vi "example_agent_example_sm_template.vi"() -> ()   [LabVIEW 2020]
uses:
  src/user_interfaces/simple_html_chat_ui/simple_html_chat_ui.lvclass
  src/models/abstract_llm_base/abstract_llm_base.lvclass
  src/vectorstore/abstract_vector_base/abstract_vector_base.lvclass
  src/agent/agent_simple_qa/agent_simple_qa.lvclass
  src/models/message_text/message_text.lvclass
  <vilib>/addons/_JKI Toolkits/State Machine/_JKI_lib_State_Machine.llb/Select State(s)_err__jki_lib_state_machine.vi
  src/vectorstore/vector_qdrant/vector_qdrant.lvclass
  C:/LV_LLM/src/vectorstore/abstract_vector_base/abstract_vector_base.lvclass
  src/models/llm_openai_chatmodels/llm_openai_chatmodels.lvclass
  C:/LV_LLM/src/models/abstract_llm_base/abstract_llm_base.lvclass
  src/models/llm_openai_embedding/llm_openai_embedding.lvclass
  src/agent/agent_simple_qa_dynamicdata/agent_simple_qa_dynamic.lvclass
  C:/LV_LLM/src/agent/agent_simple_qa/agent_simple_qa.lvclass
  <vilib>/addons/_JKI Toolkits/State Machine/_JKI_lib_State_Machine.llb/Periodic Trigger__ogtk__JKI-SM__jki_lib_state_machine.vi
  src/models/message_text/create_text_message.vi
  src/models/message_text/create_error_message.vi
  src/models/llm_openai_chatmodels/Instantiate_llm_openai.vi
  src/models/llm_openai_embedding/Instantiate_llm_openai_embed.vi
  src/agent/agent_simple_qa/poly/ask_your_data.vi
panel:
  in  "Simulate Error":bool
  in  "new_message":string
  in  "send":bool
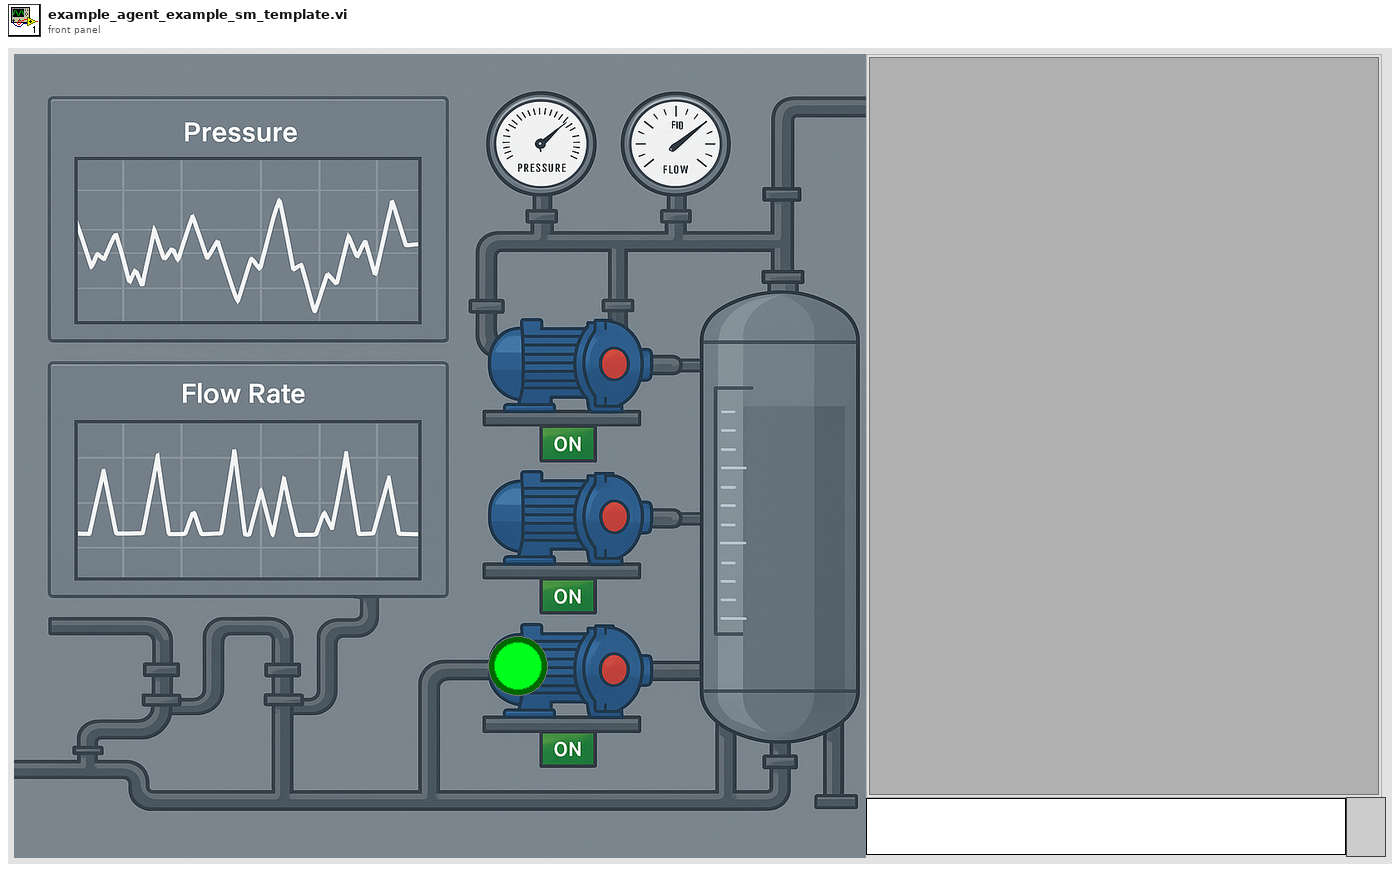
[diagram p1: front panel]
types:
  T1 = enum32{"Invalid", "Standard", "Closed", "Hidden", "Minimized", "Maximized"}
  T2 = enum32{"invalid app kind", "Development System", "Run Time System", "Student Edition", "Embedded LabVIEW", "Evaluation", "Custom"}
  T3 = cluster{"Core":cluster{"Current VI Reference":refnum<vi>, "Close Panel on Exit?":bool}, "Agent":cluster{"UI_Chat":refnum<class "simple_html_chat_ui.lvclass">, "Model_Generative":refnum<class "abstract_llm_base.lvclass">, "Model_Embedding":refnum<class "abstract_llm_base.lvclass">, "Vector Store":refnum<class "abstract_vector_base.lvclass">, "Agent_QA":refnum<class "agent_simple_qa.lvclass">, "last_message":refnum<class "message_text.lvclass">}}
  T4 = cluster{"UI_Chat":refnum<class "simple_html_chat_ui.lvclass">, "Model_Generative":refnum<class "abstract_llm_base.lvclass">, "Model_Embedding":refnum<class "abstract_llm_base.lvclass">, "Vector Store":refnum<class "abstract_vector_base.lvclass">, "Agent_QA":refnum<class "agent_simple_qa.lvclass">, "last_message":refnum<class "message_text.lvclass">}
  T5 = cluster{"Current VI Reference":refnum<vi>, "Close Panel on Exit?":bool}
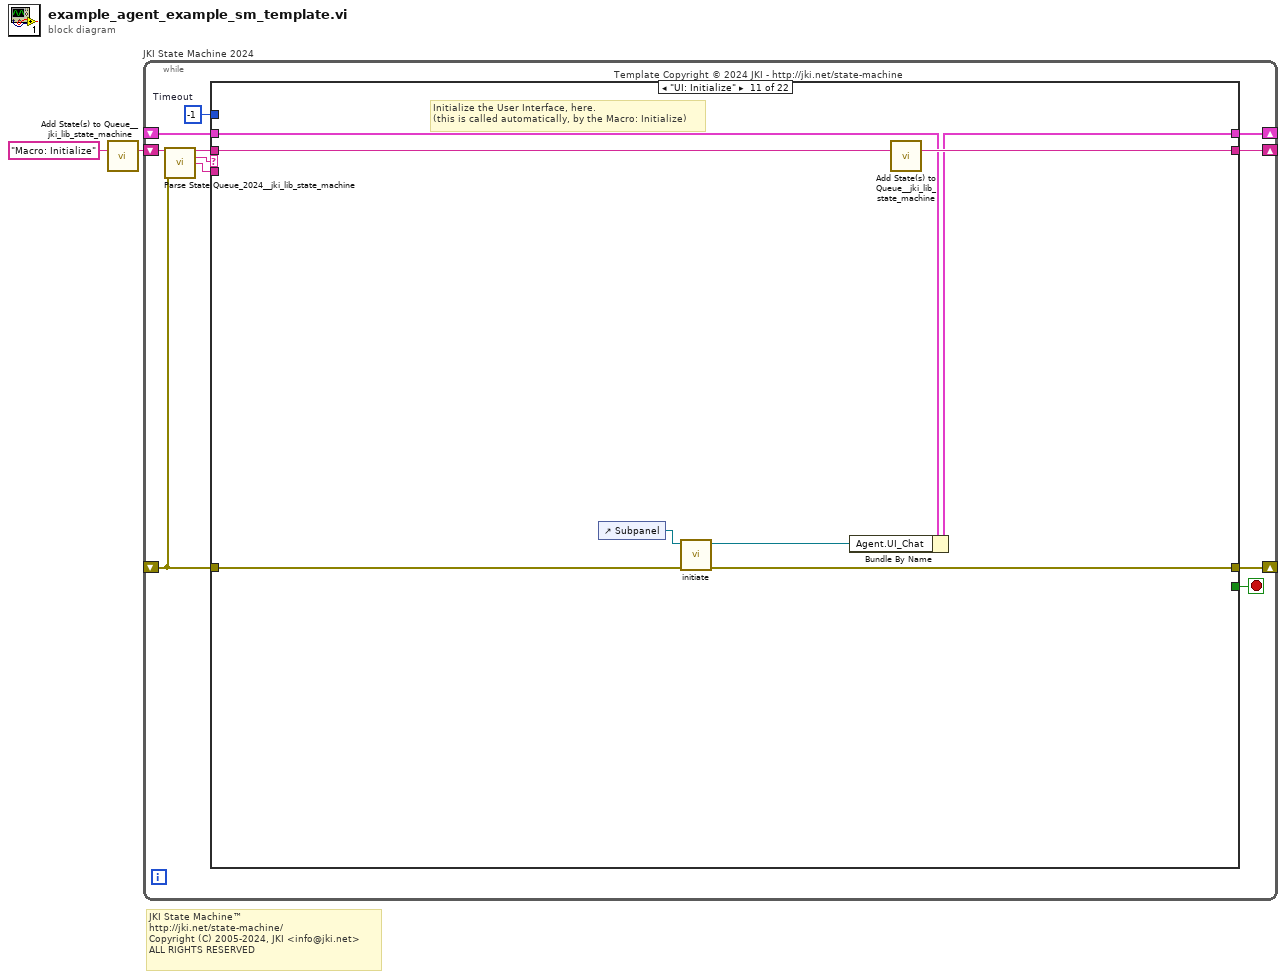
[diagram p0: block diagram]
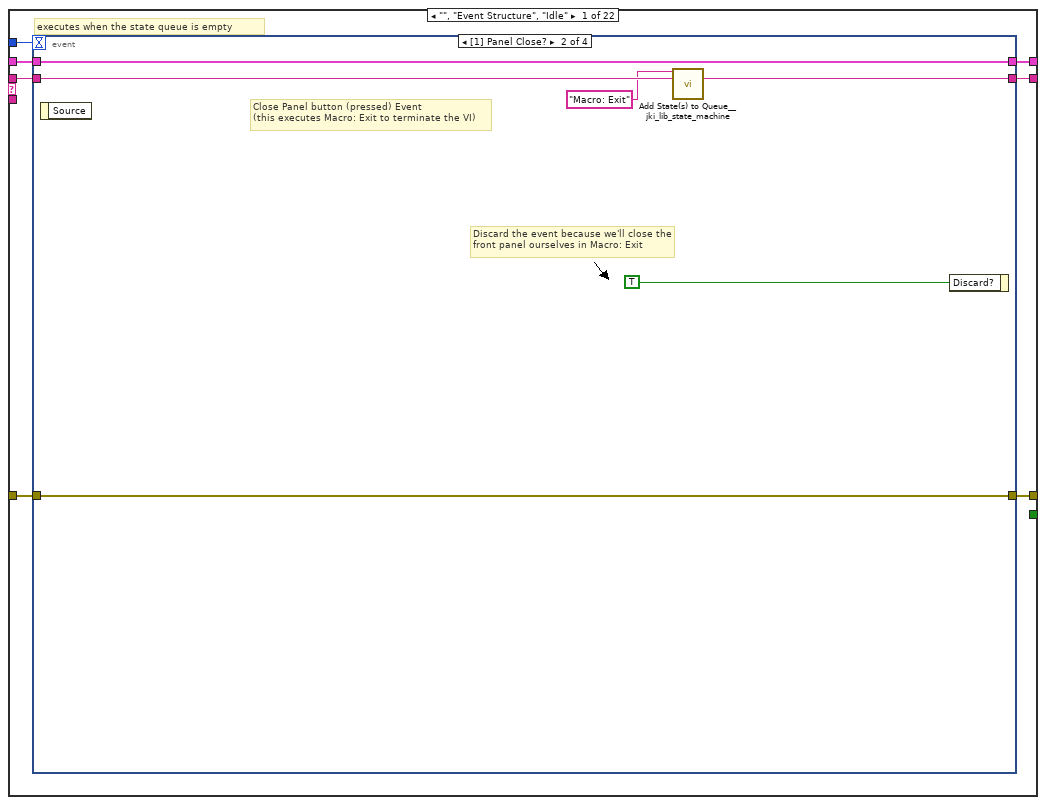
[diagram p2: hidden frame]
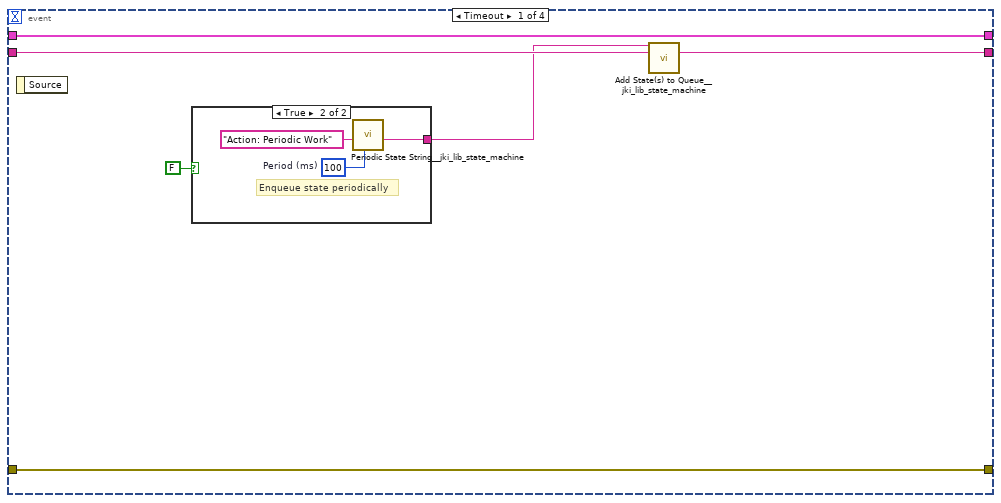
[diagram p3: hidden frame]
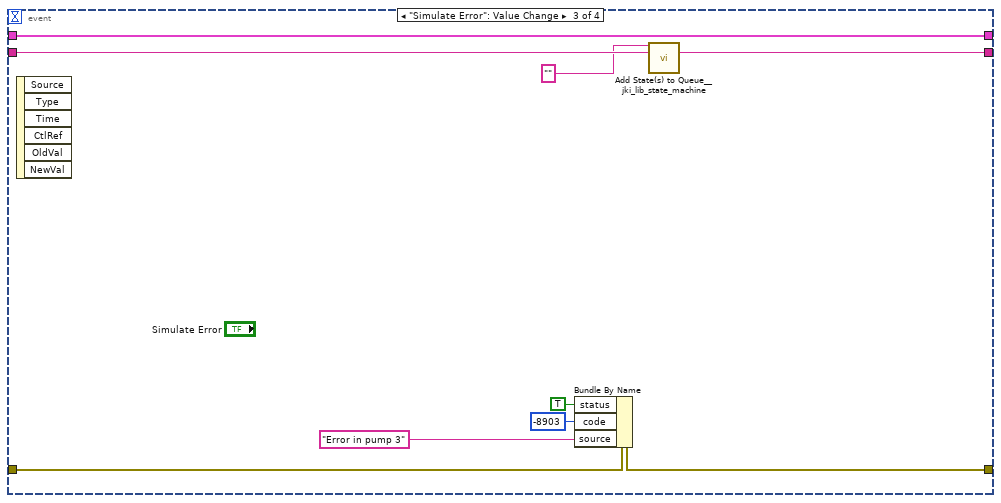
[diagram p5: hidden frame]
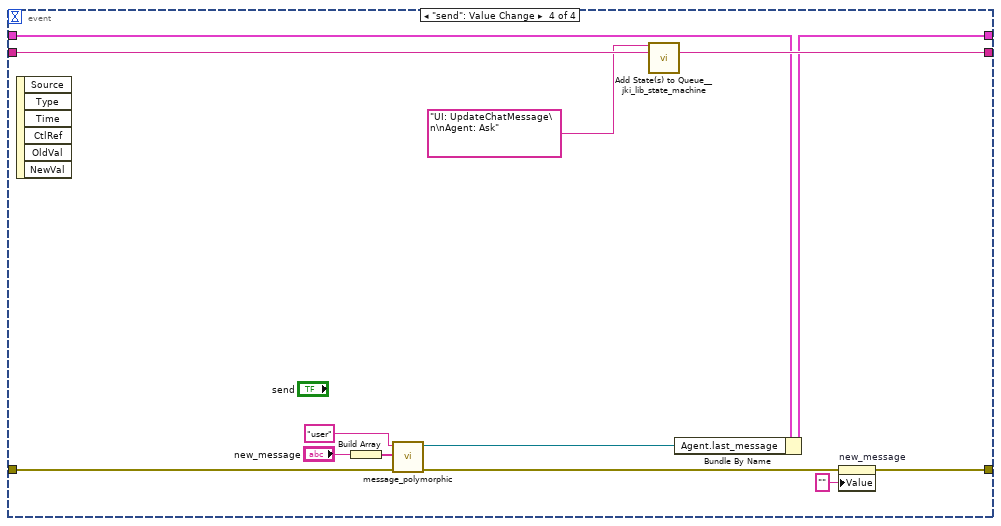
[diagram p6: hidden frame]
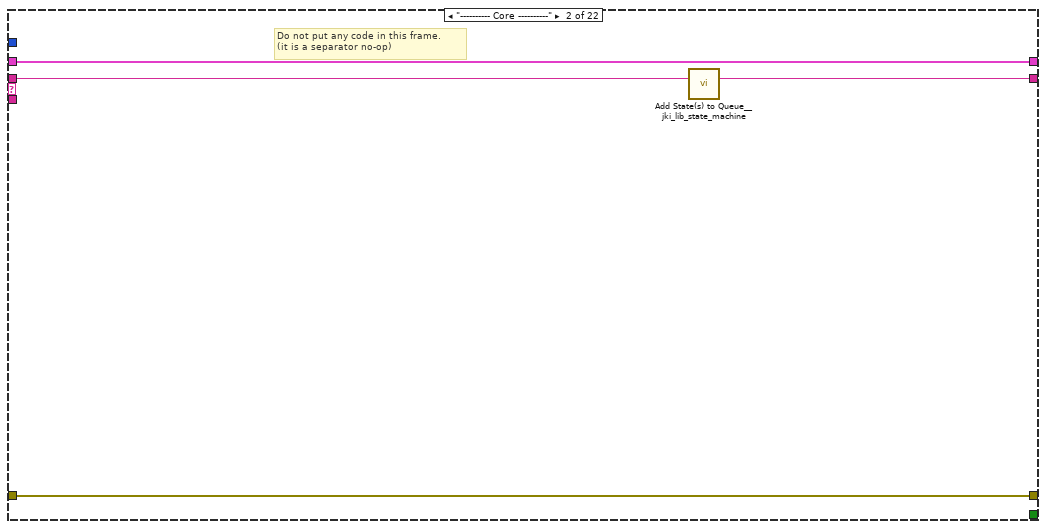
[diagram p7: hidden frame]
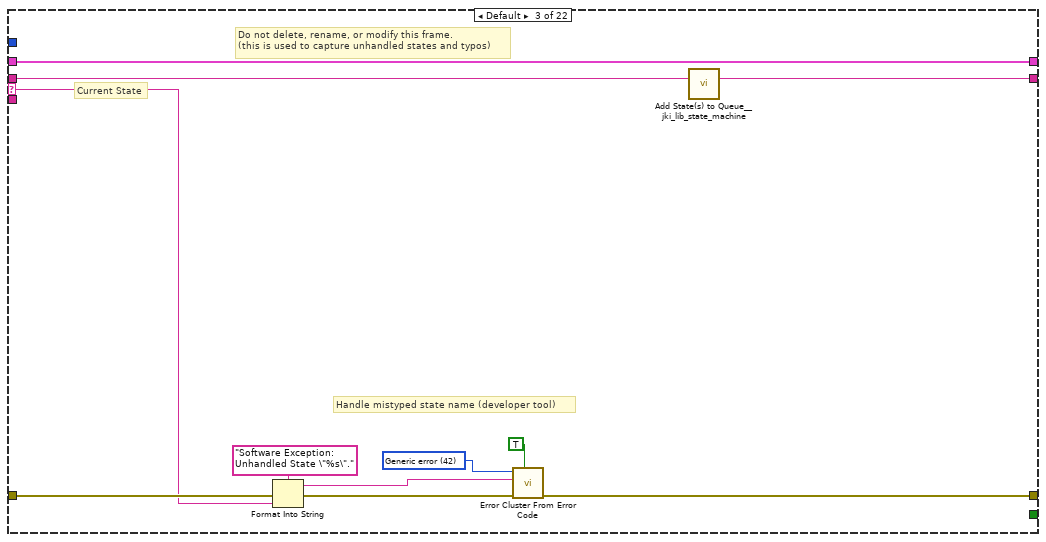
[diagram p8: hidden frame]
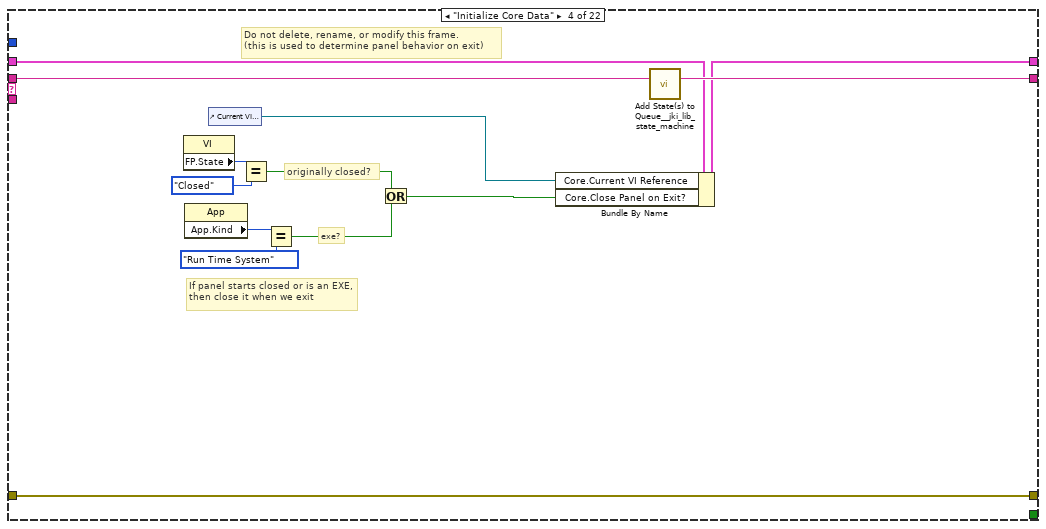
[diagram p9: hidden frame]
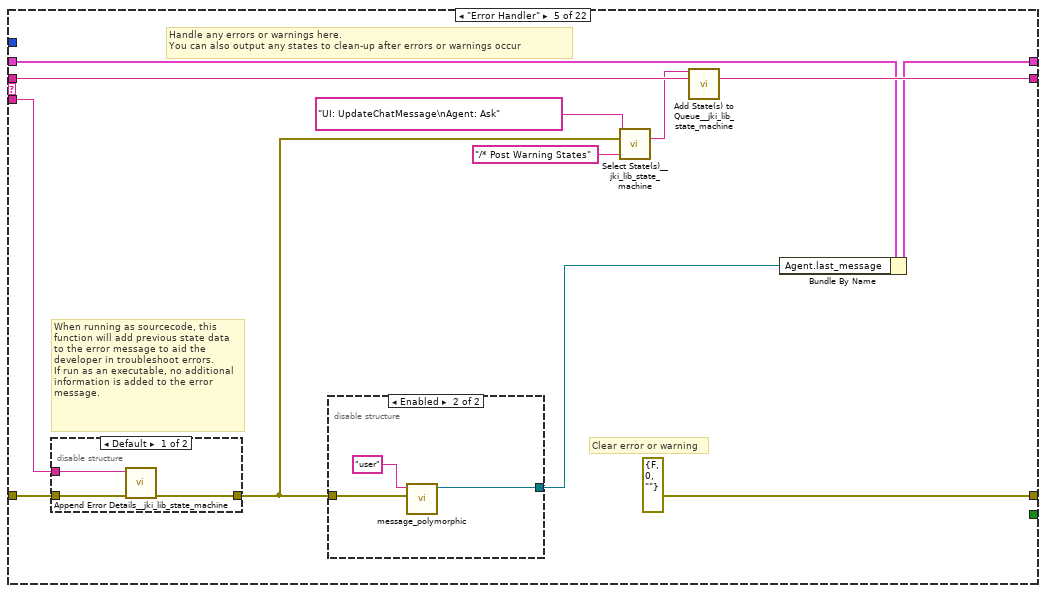
[diagram p10: hidden frame]
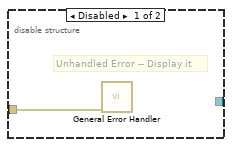
[diagram p11: hidden frame]
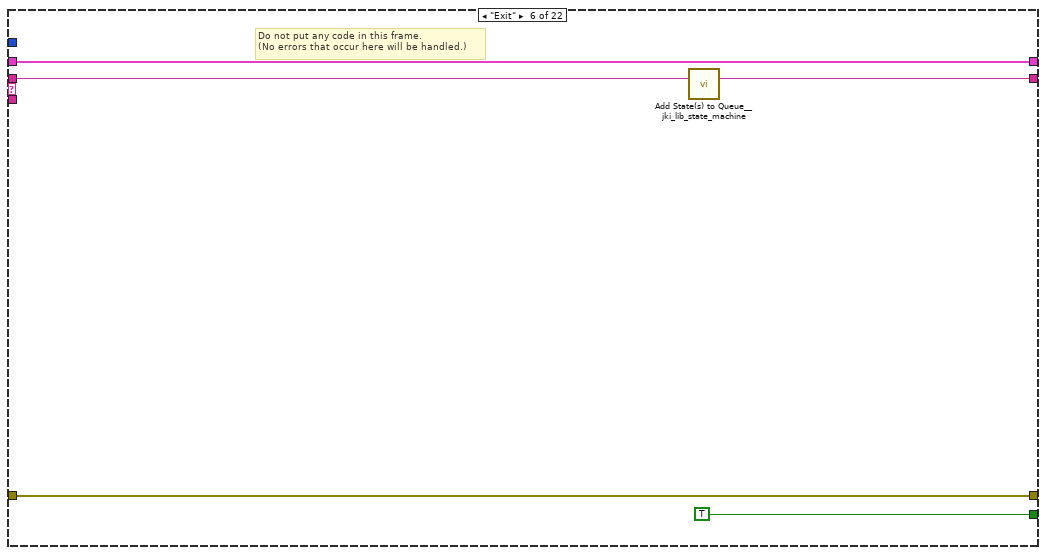
[diagram p13: hidden frame]
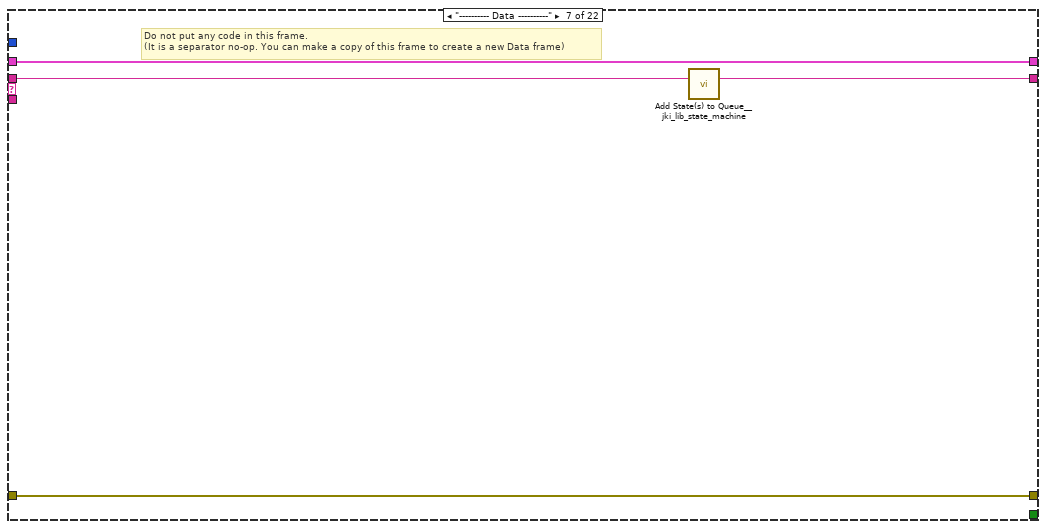
[diagram p14: hidden frame]
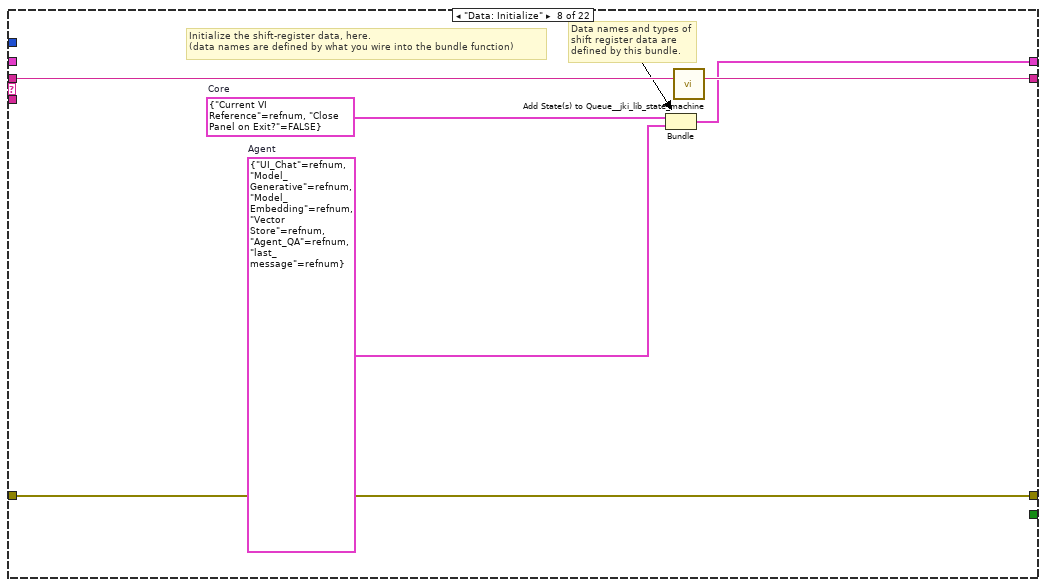
[diagram p15: hidden frame]
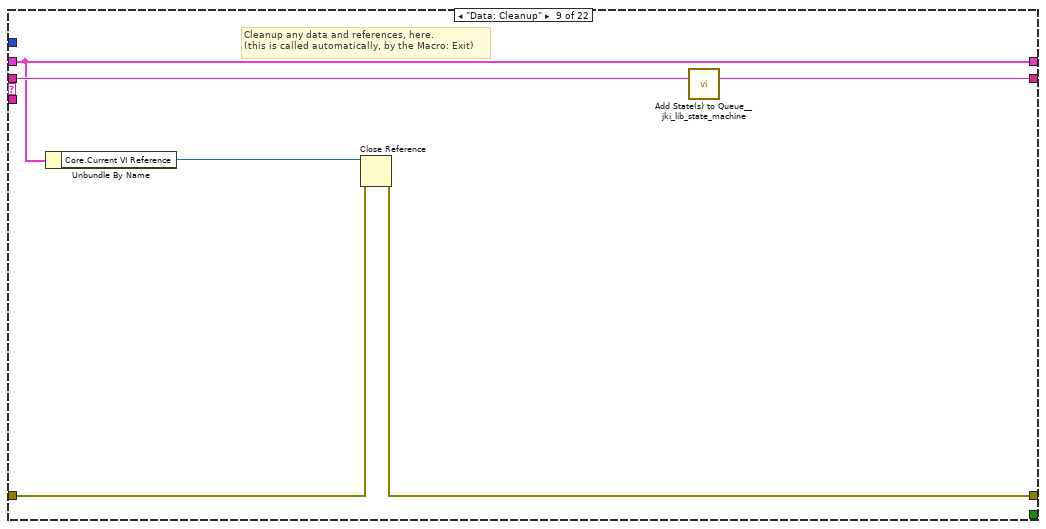
[diagram p16: hidden frame]
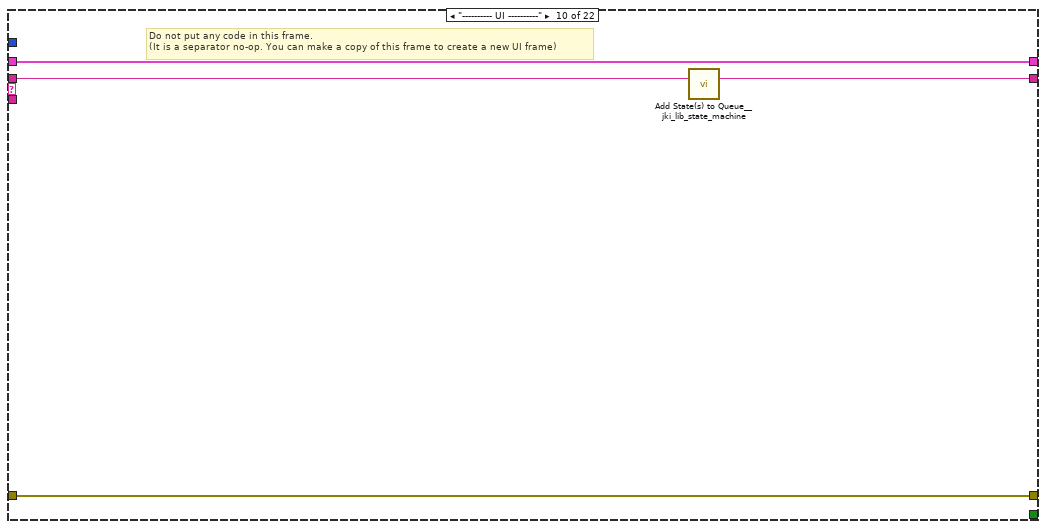
[diagram p17: hidden frame]
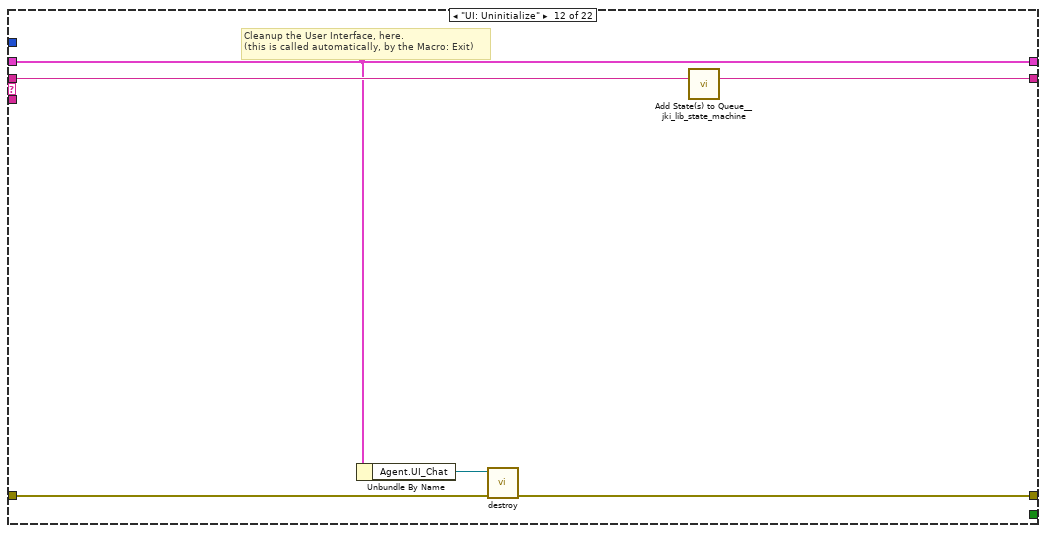
[diagram p18: hidden frame]
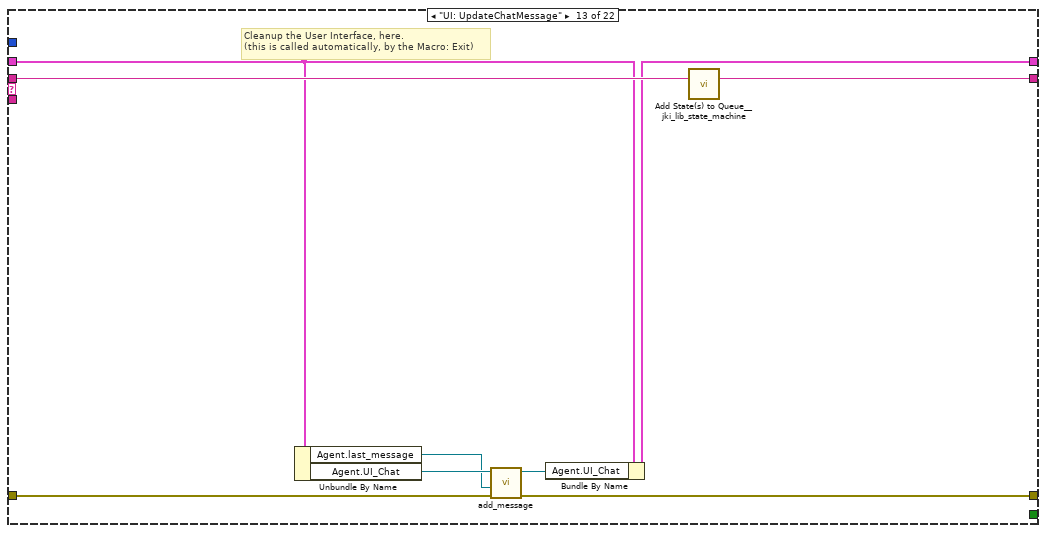
[diagram p19: hidden frame]
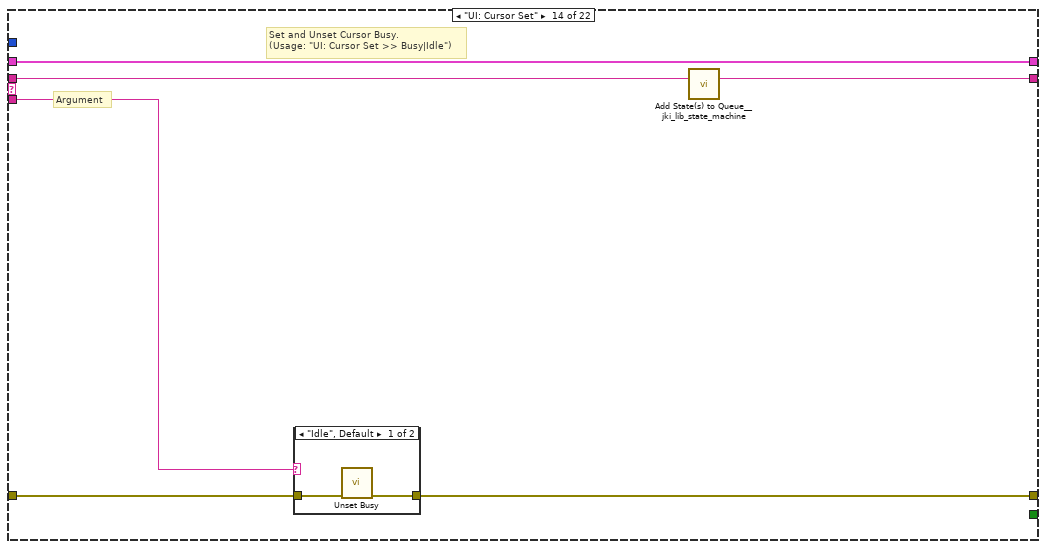
[diagram p20: hidden frame]
diagram:
  # "JKI State Machine™\nhttp://jki.net/state-machine/\nCopyright (C) 2005-2024, JKI <info@jki.net>\nALL RIGHTS RESERVED"
  n1 = call <vilib>:"Add State(s) to Queue__jki_lib_state_machine.vi"("State(s) in (\"\")"="Macro: Initialize") -> ("States Out"=w2:string)  [unwired: 14 in]
  n2 = while "JKI State Machine 2024" {
    shift-right: [w6] -> _
    shift-left: _ -> [w5]
    shift-right: [w9] -> _
    shift-left: _ -> [w3]
    shift-right: [w8] -> _
    shift-left: w2 -> [w10]
    stop <- w7 stop-if-true
    w4 = -1  # Timeout
    # "Template Copyright © 2024 JKI - http://jki.net/state-machine"
    n3 = call <vilib>:"Parse State Queue_2024__jki_lib_state_machine.vi"("State Queue"=w10, "Error In (no error)"=w3) -> ("Remaining States"=w12:string, "Current State"=w13:string, "Arguments"=w11:string)  [unwired: 11 in]
    n4 = case shown="\"UI: Initialize\"" w13 {
      selector: w13 -> [_ _ w62 _ _ _ _ _ _ _ _ _ _ _ _ _ _ _ _ _ _ _]
      tunnel: w12 -> [w20 w61 w66 w85 w97 w110 w114 w120 w126 w130 w138 w144 w153 w159 w170 w239 w244 w253 w257 w281 w293 w304]
      tunnel: w11 -> [_ _ _ _ w93 _ _ _ _ _ _ _ _ w154 w164 _ _ _ _ _ _ _]
      tunnel: w5 -> [w18 w58 w64 w78 w88 w108 w111 _ w121 w127 w133 w142 w148 w157 w166 w236 w241 w251 w254 w263 w291 w299]
      tunnel: [w17 w59 w68 w82 errorcluster {"status"=FALSE, "code"=0, "source"=""} ("error out") w107 w112 w117 w122 w128 w136 w140 w150 w155 w167 w237 w242 w248 w255 w269 w285 w300] -> w9
      tunnel: w3 -> [w14 w59 w67 w82 w94 w107 w112 w117 w123 w128 w134 w141 w151 w156 w168 w237 w242 w248 w255 w267 w289 w301]
      tunnel: [w19 w60 w65 w84 w96 w109 w113 w119 w125 w129 w137 w143 w152 w158 w169 w238 w243 w252 w256 w280 w292 w303] -> w8
      tunnel: [_ _ _ _ _ TRUE _ _ _ _ _ _ _ _ _ _ _ _ _ _ _ _] -> w7
      tunnel: [w16 w58 w64 w83 w86 w108 w111 w118 w121 w127 w132 w142 w147 w157 w166 w236 w241 w251 w254 w262 w291 w297] -> w6
      tunnel: w4 -> [w15 _ _ _ _ _ _ _ _ _ _ _ _ _ _ _ _ _ _ _ _ _]
      frame "", "Event Structure", "Idle" {
        # "executes when the state queue is empty"
        n5 = event shown="[1] Panel Close?" {
          selector: _ -> [_ _ _ _]
          dyn-events: _ -> [_ _ _ _]
          timeout: w15 -> [_ _ _ _]
          tunnel: w20 -> [w26 w35 w44 w57]
          tunnel: [w25 w34 w43 w56] -> w19
          tunnel: w18 -> [w23 w32 w42 w50]
          tunnel: [w24 w33 w39 w46] -> w17
          tunnel: w14 -> [w24 w33 w40 w52]
          tunnel: [w23 w32 w42 w48] -> w16
          event Timeout {
            n6 = event-data() -> ()  [unwired: 1 in, 1 out]
            n7 = case shown="True" FALSE {
              tunnel: [_ w29] -> w22
              frame False {
              }
              frame True {
                w27 = u32 100  # Period (ms)
                # "Enqueue state periodically"
                n8 = call <vilib>:"Periodic State String__jki_lib_state_machine.vi"("Period (ms)"=w27, "State"="Action: Periodic Work") -> ("State Out"=w29:string)  [unwired: 9 in]
              }
            }
            n9 = call <vilib>:"Add State(s) to Queue__jki_lib_state_machine.vi"("State(s) in Front (\"\")"=w22, "State(s) in (\"\")"=w26) -> ("States Out"=w25:string)  [unwired: 13 in]
          }
          event Panel Close? {
            # "Discard the event because we'll close the front panel ourselves in Macro: Exit"
            # "Close Panel button (pressed) Event\n(this executes Macro: Exit to terminate the VI)"
            n10 = event-data() -> ()  [unwired: 1 in, 1 out]
            n11 = call <vilib>:"Add State(s) to Queue__jki_lib_state_machine.vi"("State(s) in Front (\"\")"="Macro: Exit", "State(s) in (\"\")"=w35) -> ("States Out"=w34:string)  [unwired: 13 in]
            n12 = event-data("Discard?"=TRUE) -> ()  [unwired: 1 in, 1 out]
          }
          event "Simulate Error": Value Change {
            n13 = event-data() -> ()  [unwired: 1 in, 6 out]
            n14 = Bundle By Name(cluster=w40, "status"=TRUE, "code"=-8903, "source"="Error in pump 3") -> (w39:errorcluster)
            n15 = call <vilib>:"Add State(s) to Queue__jki_lib_state_machine.vi"("State(s) in Front (\"\")"="", "State(s) in (\"\")"=w44) -> ("States Out"=w43:string)  [unwired: 13 in]
          }
          event "send": Value Change {
            n16 = event-data() -> ()  [unwired: 1 in, 6 out]
            n17 = Build Array("new_message") -> (w53:string[])
            n18 = call-poly "message_polymorphic.vi"("error in (no error)"=w52, "content"=w53, "role"="user") -> ("error out"=w47:errorcluster, "message_text out"=w49:refnum<class "message_text.lvclass">)  [unwired: 7 in]
            n19 = call <vilib>:"Add State(s) to Queue__jki_lib_state_machine.vi"("State(s) in Front (\"\")"="UI: UpdateChatMessage\n\nAgent: Ask", "State(s) in (\"\")"=w57) -> ("States Out"=w56:string)  [unwired: 13 in]
            n20 = Bundle By Name(cluster=w50, "Agent.last_message"=w49) -> (w48:T3)
            n21 = property on="new_message" class="Str"(error in=w47, "Value"="" ("new_message")) -> (error out=w46:errorcluster)  [unwired: 1 in, 1 out]
          }
        }
      }
      frame "---------- Core ----------" {
        # "Do not put any code in this frame.\n(it is a separator no-op)"
        n22 = call <vilib>:"Add State(s) to Queue__jki_lib_state_machine.vi"("State(s) in (\"\")"=w61) -> ("States Out"=w60:string)  [unwired: 14 in]
      }
      frame Default {
        w71 = 42 items=["No error", "Argument error", "Memory is full", "Out of zone", "End of file", "File already open", "Generic file I/O error", "File not found", "File permission error", "Disk is full", "Duplicate path", "Too many files open", "System feature not enabled", "Resource file not found", "Cannot add resource", "Resource not found", "Image not found", "Image memory error", "Pen does not exist", "Config type invalid", "Config token not found", "Config parse error", "Config memory error", "Bad external code format", "Bad external code offset", "External code not present", "Null window", "Destroy window error", "Null menu", "Print aborted", "Bad print record", "Print driver error", "Windows error during printing", "Memory error during printing", "Print dialog error", "Generic print error", "Invalid device refnum", "Device not found", "Device parameter error", "Device unit error", "Cannot open device", "Device call aborted", "Generic error", "Cancelled by user", "Object ID too low", "Object ID too high", "Object not in heap", "Unknown heap", "Unknown object (invalid DefProc)", "Unknown object (DefProc not in table)", "Message out of range", "Invalid (null) method", "Unknown message", "Manager call not supported", "Bad address", "Network operation in progress", "Network operation timed out", "Connection is busy", "Network attribute not supported", "Network error", "Address in use", "System out of memory", "Connection aborted", "Connection refused", "Not connected", "Already connected", "Connection closed", "Initialization error (interapplication manager)", "Bad occurrence", "Wait on unbound occurrence handler", "Occurrence queue overflow", "Datalog type conflict", "Unused", "Unrecognized type (interapplication manager)", "Memory corrupt", "Failed to make temporary DLL", "Old CIN version", "Drag socket not found", "Failed to load drop-object", "Failed to register OLE object", "Failed to release OLE object", "Format specifier type mismatch", "Unknown format specifier", "Too few format specifiers", "Too many format specifiers", "Scan failed", "Newer CIN version", "Error converting to variant", "Runtime menu error", "Password tampered", "Variant attribute not found", "Incompatible variant data type", "Event data is not available", "Event Store is not present", "Occurrence is not found", "Event Queue is not created", "Event info is not available", "Refnum passed is NULL", "Error retrieving Class GUID", "Error retrieving CoClass GUID", "Error retrieving TypeLib GUID.", "Bad built application magic bytes.", "Specific driver is different from the specific driver associated with the Logical Name.", "There is no session opened to the class driver.", "Max Error", "MAX - Error with config objects", "MAX - Error loading configuration", "MAX - Group not supported"]
        # "Current State"
        # "Do not delete, rename, or modify this frame.\n(this is used to capture unhandled states and typos)"
        # "Handle mistyped state name (developer tool)"
        n23 = Format Into String(format string="Software Exception: Unhandled State \"%s\"." ("message"), error in=w67, w62) -> (resulting string=w70:string, error out=w69:errorcluster)  [unwired: 1 in]
        n24 = call <vilib>:"Error Cluster From Error Code.vi"("show call chain? (False)"=TRUE, "error in (no error)"=w69, "error message (\"\")"=w70, "error code (0)"=w71) -> ("error out"=w68:errorcluster)  [unwired: 5 in]
        n25 = call <vilib>:"Add State(s) to Queue__jki_lib_state_machine.vi"("State(s) in (\"\")"=w66) -> ("States Out"=w65:string)  [unwired: 14 in]
      }
      frame "Initialize Core Data" {
        # "Do not delete, rename, or modify this frame.\n(this is used to determine panel behavior on exit)"
        # "originally closed?"
        # "exe?"
        # "If panel starts closed or is an EXE, then close it when we exit"
        n26 = property class="VI"() -> ("FP.State"=w75:T1)  [unwired: 2 in, 2 out]
        n27 = property class="App"() -> ("App.Kind"=w81:T2)  [unwired: 2 in, 2 out]
        n28 = control-ref of="Current VI Reference"() -> (w76:refnum<vi>)
        n29 = Equal?(x=w75, y=T1."Closed" ("Front Panel Window:State")) -> (x = y?=w73:bool)
        n30 = Equal?(x=w81, y=T2."Run Time System" ("Application:Kind")) -> (x = y?=w79:bool)
        n31 = Or(x=w73, y=w79) -> (x .or. y?=w77:bool)
        n32 = Bundle By Name(cluster=w78, "Core.Current VI Reference"=w76, "Core.Close Panel on Exit?"=w77) -> (w83:T3)
        n33 = call <vilib>:"Add State(s) to Queue__jki_lib_state_machine.vi"("State(s) in (\"\")"=w85) -> ("States Out"=w84:string)  [unwired: 14 in]
      }
      frame "Error Handler" {
        # "When running as sourcecode, this function will add previous state data to the error message to aid the developer in troubleshoot errors.\nIf run as an executable, no additional information is added to the error message."
        # "Handle any errors or warnings here.\nYou can also output any states to clean-up after errors or warnings occur"
        # "Clear error or warning"
        n34 = disable-structure shown="Default" {
          disable-tunnel: w94 -> [w104 w105]
          disable-tunnel: w93 -> [w103 _]
          disable-tunnel: [w102 w105] -> w92
          frame condition #0 (active) {
            n35 = call <vilib>:"Append Error Details__jki_lib_state_machine.vi"("error in (no error)"=w104, "Previous State and Argument(s)"=w103) -> ("error out"=w102:errorcluster)  [unwired: 9 in]
          }
          frame condition #1 {
          }
        }
        n36 = disable-structure shown="Enabled" {
          disable-tunnel: w92 -> [w98 w99]
          disable-tunnel: [_ w100] -> w87
          frame Disabled {
            # "Unhandled Error -- Display it"
            n37 = call <vilib>:"General Error Handler.vi"("error in (no error)"=w98) -> ()  [unwired: 10 in, 5 out]
          }
          frame Enabled {
            n38 = call-poly "message_polymorphic.vi"("Error Message"=w99, "role"="user") -> ("message_text out"=w100:refnum<class "message_text.lvclass">)  [unwired: 8 in, 1 out]
          }
        }
        n39 = call-poly <vilib>:"Select State(s)__jki_lib_state_machine.vi"("State(s) if True (\"\")"="UI: UpdateChatMessage\nAgent: Ask", "Select"=w92, "State(s) if False (\"\")"="/* Post Warning States") -> ("States Out"=w90:string)  [unwired: 12 in]
        n40 = call <vilib>:"Add State(s) to Queue__jki_lib_state_machine.vi"("State(s) in Front (\"\")"=w90, "State(s) in (\"\")"=w97) -> ("States Out"=w96:string)  [unwired: 13 in]
        n41 = Bundle By Name(cluster=w88, "Agent.last_message"=w87) -> (w86:T3)
      }
      frame "Exit" {
        # "Do not put any code in this frame.\n(No errors that occur here will be handled.)"
        n42 = call <vilib>:"Add State(s) to Queue__jki_lib_state_machine.vi"("State(s) in (\"\")"=w110) -> ("States Out"=w109:string)  [unwired: 14 in]
      }
      frame "---------- Data ----------" {
        # "Do not put any code in this frame.\n(It is a separator no-op. You can make a copy of this frame to create a new Data frame)"
        n43 = call <vilib>:"Add State(s) to Queue__jki_lib_state_machine.vi"("State(s) in (\"\")"=w114) -> ("States Out"=w113:string)  [unwired: 14 in]
      }
      frame "Data: Initialize" {
        w115 = T4 {"UI_Chat"=refnum, "Model_Generative"=refnum, "Model_Embedding"=refnum, "Vector Store"=refnum, "Agent_QA"=refnum, "last_message"=refnum}  # Agent
        w116 = T5 {"Current VI Reference"=refnum, "Close Panel on Exit?"=FALSE}  # Core
        # "Data names and types of shift register data are defined by this bundle."
        # "Initialize the shift-register data, here.\n(data names are defined by what you wire into the bundle function)"
        n44 = Bundle("Core"=w116, "Agent"=w115) -> (w118:T3)  [unwired: 1 in]
        n45 = call <vilib>:"Add State(s) to Queue__jki_lib_state_machine.vi"("State(s) in (\"\")"=w120) -> ("States Out"=w119:string)  [unwired: 14 in]
      }
      frame "Data: Cleanup" {
        # "Cleanup any data and references, here.\n(this is called automatically, by the Macro: Exit)"
        n46 = Unbundle By Name(w121) -> ("Core.Current VI Reference"=w124:refnum<vi>)
        n47 = Close Reference(reference=w124, error in (no error)=w123) -> (error out=w122:errorcluster)
        n48 = call <vilib>:"Add State(s) to Queue__jki_lib_state_machine.vi"("State(s) in (\"\")"=w126) -> ("States Out"=w125:string)  [unwired: 14 in]
      }
      frame "---------- UI ----------" {
        # "Do not put any code in this frame.\n(It is a separator no-op. You can make a copy of this frame to create a new UI frame)"
        n49 = call <vilib>:"Add State(s) to Queue__jki_lib_state_machine.vi"("State(s) in (\"\")"=w130) -> ("States Out"=w129:string)  [unwired: 14 in]
      }
      frame "UI: Initialize" {
        # "Initialize the User Interface, here.\n(this is called automatically, by the Macro: Initialize)"
        n50 = control-ref of="Subpanel"() -> (w131:refnum<vi>)
        n51 = call "initiate.vi"("error in"=w134, "Sub Panel"=w131) -> ("error out"=w136:errorcluster, "simple_html_chat_ui out"=w135:refnum<class "simple_html_chat_ui.lvclass">)  [unwired: 8 in]
        n52 = Bundle By Name(cluster=w133, "Agent.UI_Chat"=w135) -> (w132:T3)
        n53 = call <vilib>:"Add State(s) to Queue__jki_lib_state_machine.vi"("State(s) in (\"\")"=w138) -> ("States Out"=w137:string)  [unwired: 14 in]
      }
      frame "UI: Uninitialize" {
        # "Cleanup the User Interface, here.\n(this is called automatically, by the Macro: Exit)"
        n54 = Unbundle By Name(w142) -> ("Agent.UI_Chat"=w139:refnum<class "simple_html_chat_ui.lvclass">)
        n55 = call "destroy.vi"("error in (no error)"=w141, "simple_html_chat_ui in"=w139) -> ("error out"=w140:errorcluster)  [unwired: 8 in, 1 out]
        n56 = call <vilib>:"Add State(s) to Queue__jki_lib_state_machine.vi"("State(s) in (\"\")"=w144) -> ("States Out"=w143:string)  [unwired: 14 in]
      }
      frame "UI: UpdateChatMessage" {
        # "Cleanup the User Interface, here.\n(this is called automatically, by the Macro: Exit)"
        n57 = Unbundle By Name(w148) -> ("Agent.last_message"=w145:refnum<class "message_text.lvclass">, "Agent.UI_Chat"=w149:refnum<class "simple_html_chat_ui.lvclass">)
        n58 = call "add_message.vi"("error in (no error)"=w151, "message_text.lvclass"=w145, "simple_html_chat_ui in"=w149) -> ("error out"=w150:errorcluster, "simple_html_chat_ui out"=w146:refnum<class "simple_html_chat_ui.lvclass">)  [unwired: 7 in]
        n59 = Bundle By Name(cluster=w148, "Agent.UI_Chat"=w146) -> (w147:T3)
        n60 = call <vilib>:"Add State(s) to Queue__jki_lib_state_machine.vi"("State(s) in (\"\")"=w153) -> ("States Out"=w152:string)  [unwired: 14 in]
      }
      frame "UI: Cursor Set" {
        # "Argument"
        # "Set and Unset Cursor Busy.\n(Usage: \"UI: Cursor Set >> Busy|Idle\")"
        n61 = case shown="\"Idle\", Default" w154 {
          tunnel: w156 -> [w161 w163]
          tunnel: [w160 w162] -> w155
          frame "Idle", Default {
            n62 = call <vilib>:"Unset Busy.vi"("error in (no error)"=w161) -> ("error out"=w160:errorcluster)  [unwired: 10 in]
          }
          frame "Busy" {
            n63 = call <vilib>:"Set Busy.vi"("error in (no error)"=w163) -> ("error out"=w162:errorcluster)  [unwired: 9 in, 1 out]
          }
        }
        n64 = call <vilib>:"Add State(s) to Queue__jki_lib_state_machine.vi"("State(s) in (\"\")"=w159) -> ("States Out"=w158:string)  [unwired: 14 in]
      }
      frame "UI: Front Panel State" {
        # "Argument"
        # "Set Front Panel Open or Closed\n(Usage: \"UI: Front Panel State >> Open|Close\")"
        n65 = Unbundle By Name(w166) -> ("Core.Current VI Reference"=w165:refnum<vi>)
        n66 = case shown="\"Minimize\", \"Minimized\"" w164 {
          tunnel: w168 -> [w176 w191 w202 w215 w228]
          tunnel: [w178 w192 w204 w217 w230] -> w167
          tunnel: w165 -> [w177 w189 w203 w216 w229]
          frame "Open", "Standard", Default {
            w171 = T1."Standard" ("State")
            n67 = property class="VI"(reference=w177, error in=w176) -> (reference out=w174:refnum<vi>, error out=w175:errorcluster, "FP.State"=w173:T1)
            n68 = Not Equal?(x=w173, y=w171) -> (x != y?=w172:bool)
            n69 = case shown="True" w172 {
              tunnel: [w182 w184] -> w178
              tunnel: w175 -> [w181 w184]
              tunnel: w174 -> [w180 _]
              tunnel: w171 -> [w179 _]
              frame True {
                n70 = invoke class="VI" method="FP.Open"(reference=w180, error in=w181, "Activate"=TRUE, "State"=w179) -> (error out=w182:errorcluster)  [unwired: 1 in, 4 out]
              }
              frame False {
              }
            }
          }
          frame "Close", "Closed" {
            n71 = property class="VI"(reference=w189, error in=w191) -> (reference out=w188:refnum<vi>, error out=w190:errorcluster, "FP.State"=w186:T1)
            n72 = Not Equal?(x=w186, y=T1."Closed" ("Front Panel Window:State")) -> (x != y?=w185:bool)
            n73 = case shown="True" w185 {
              tunnel: [w193 w196] -> w192
              tunnel: w190 -> [w193 w195]
              tunnel: w188 -> [_ w194]
              frame False {
              }
              frame True {
                n74 = invoke class="VI" method="FP.Close"(reference=w194, error in=w195) -> (error out=w196:errorcluster)  [unwired: 1 in, 2 out]
              }
            }
          }
          frame "Hidden", "Hide" {
            w197 = T1."Hidden" ("State")
            n75 = property class="VI"(reference=w203, error in=w202) -> (reference out=w200:refnum<vi>, error out=w201:errorcluster, "FP.State"=w199:T1)
            n76 = Not Equal?(x=w199, y=w197) -> (x != y?=w198:bool)
            n77 = case shown="True" w198 {
              tunnel: [w208 w209] -> w204
              tunnel: w201 -> [w207 w209]
              tunnel: w200 -> [w206 _]
              tunnel: w197 -> [w205 _]
              frame True {
                n78 = invoke class="VI" method="FP.Open"(reference=w206, error in=w207, "State"=w205) -> (error out=w208:errorcluster)  [unwired: 2 in, 4 out]
              }
              frame False {
              }
            }
          }
          frame "Minimize", "Minimized" {
            w210 = T1."Minimized" ("State")
            n79 = property class="VI"(reference=w216, error in=w215) -> (reference out=w213:refnum<vi>, error out=w214:errorcluster, "FP.State"=w212:T1)
            n80 = Not Equal?(x=w212, y=w210) -> (x != y?=w211:bool)
            n81 = case shown="True" w211 {
              tunnel: [w221 w222] -> w217
              tunnel: w214 -> [w220 w222]
              tunnel: w213 -> [w219 _]
              tunnel: w210 -> [w218 _]
              frame True {
                n82 = invoke class="VI" method="FP.Open"(reference=w219, error in=w220, "State"=w218) -> (error out=w221:errorcluster)  [unwired: 2 in, 4 out]
              }
              frame False {
              }
            }
          }
          frame "Maximize", "Maximized" {
            w223 = T1."Maximized" ("State")
            n83 = property class="VI"(reference=w229, error in=w228) -> (reference out=w226:refnum<vi>, error out=w227:errorcluster, "FP.State"=w225:T1)
            n84 = Not Equal?(x=w225, y=w223) -> (x != y?=w224:bool)
            n85 = case shown="True" w224 {
              tunnel: [w234 w235] -> w230
              tunnel: w227 -> [w233 w235]
              tunnel: w226 -> [w232 _]
              tunnel: w223 -> [w231 _]
              frame True {
                n86 = invoke class="VI" method="FP.Open"(reference=w232, error in=w233, "State"=w231) -> (error out=w234:errorcluster)  [unwired: 2 in, 4 out]
              }
              frame False {
              }
            }
          }
        }
        n87 = call <vilib>:"Add State(s) to Queue__jki_lib_state_machine.vi"("State(s) in (\"\")"=w170) -> ("States Out"=w169:string)  [unwired: 14 in]
      }
      frame "---------- Macro ----------" {
        # "Do not put any code in this frame.\n(It is a separator no-op. You can make a copy of this frame to create a new Macro frame)"
        n88 = call <vilib>:"Add State(s) to Queue__jki_lib_state_machine.vi"("State(s) in (\"\")"=w239) -> ("States Out"=w238:string)  [unwired: 14 in]
      }
      frame "Macro: Initialize" {
        w240 = "Data: Initialize\nInitialize Core Data\nUI: Initialize\nUI: Front Panel State >> Open\n\nAgent: Initialize"  # Data: Initialize Initialize Core Data UI: Initialize UI: Front Panel State >> Open  Agent: Initialize
        # "Initialization Macro\n(This is called once, when the VI starts)"
        n89 = call <vilib>:"Add State(s) to Queue__jki_lib_state_machine.vi"("State(s) in Front (\"\")"=w240, "State(s) in (\"\")"=w244) -> ("States Out"=w243:string)  [unwired: 13 in]
      }
      frame "Macro: Exit" {
        # "Exit Macro\n(This is called once, when the VI exits)"
        n90 = Unbundle By Name(w251) -> ("Core.Close Panel on Exit?"=w246:bool)
        n91 = call <vilib>:"Conditional State String__jki_lib_state_machine.vi"("Do State(s)?"=w246, "State"="UI: Front Panel State >> Close") -> ("State Out"=w245:string)  [unwired: 7 in]
        n92 = call <vilib>:"Add State(s) to Queue__jki_lib_state_machine.vi"("State(s) in (\"\")"=w245, "State(s) at Back (\"\")"="UI: Uninitialize\nData: Cleanup\n\nAgent: Close\n\nExit") -> ("States Out"=w249:string)  [unwired: 13 in]
        n93 = call <vilib>:"Add State(s) to Queue__jki_lib_state_machine.vi"("State(s) in Front (\"\")"=w249, "State(s) in (\"\")"=w253) -> ("States Out"=w252:string)  [unwired: 13 in]
      }
      frame "----------Agents----------" {
        # "Template Separator\n(You can make a copy of, or modify, this frame)"
        n94 = call <vilib>:"Add State(s) to Queue__jki_lib_state_machine.vi"("State(s) in (\"\")"=w257) -> ("States Out"=w256:string)  [unwired: 14 in]
      }
      frame "Agent: Initialize" {
        w270 = FALSE  # skip_loading_data
        # "Your code here.\n(You can make a copy of, or modify, this frame)"
        n95 = call "get_env_variable.vi"("Environment Variable Name"="labview_llm_openai_key") -> ("Value"=w277:string)  [unwired: 1 in, 1 out]
        n96 = call "get_env_variable.vi"("Environment Variable Name"="labview_llm_openai_key") -> ("Value"=w272:string)  [unwired: 1 in, 1 out]
        n97 = call "instantiate_qdrant_vector.vi"("host_url"="http://10.0.0.209:6333/", "error in"=w267) -> ("vector_qdrant out"=w260:refnum<class "vector_qdrant.lvclass">, "error out"=w265:errorcluster)  [unwired: 12 in]
        n98 = call-poly "instantiate_chat_model.vi"("model_name"="gpt-4o-mini", "openai_key"=w277, "error in (no error)"=w267) -> ("llm_openai out"=w259:refnum<class "llm_openai_chatmodels.lvclass">, "error out"=w264:errorcluster)  [unwired: 11 in]
        n99 = call-poly "instantiate_embedding_model.vi"("model_name"="text-embedding-ada-002", "openai_key"=w272, "error in (no error)"=w267) -> ("llm_openai_embedding out"=w258:refnum<class "llm_openai_embedding.lvclass">, "error out"=w268:errorcluster)  [unwired: 11 in]
        n100 = Merge Errors(w265, w264, w268) -> (w266:errorcluster)
        n101 = call "instantiate_simple_qa_dynamic.vi"("vectorestore"=w260, "skip_loading_data"=w270, "collection_name"="example_pipeline_collection" ("host_url"), "chat_model"=w259, "embedding_model"=w258, "error in (no error)"=w266, "sources"=string[] [] ("webpages")) -> ("agent_webpage_qa out"=w261:refnum<class "agent_simple_qa_dynamic.lvclass">, "error out"=w269:errorcluster)  [unwired: 7 in]
        n102 = call <vilib>:"Add State(s) to Queue__jki_lib_state_machine.vi"("State(s) in (\"\")"=w281) -> ("States Out"=w280:string)  [unwired: 14 in]
        n103 = Bundle By Name(cluster=w263, "Agent.Vector Store"=w260, "Agent.Model_Generative"=w259, "Agent.Model_Embedding"=w258, "Agent.Agent_QA"=w261) -> (w262:T3)
      }
      frame "Agent: Close" {
        # "Your code here.\n(You can make a copy of, or modify, this frame)"
        n104 = Unbundle By Name(w291) -> ("Agent.Model_Generative"=w282:refnum<class "abstract_llm_base.lvclass">, "Agent.Model_Embedding"=w283:refnum<class "abstract_llm_base.lvclass">, "Agent.Vector Store"=w284:refnum<class "abstract_vector_base.lvclass">, "Agent.Agent_QA"=w290:refnum<class "agent_simple_qa.lvclass">)
        n105 = call-dynamic "destroy.vi"("agent_simple_qa in"=w290, "error in (no error)"=w289) -> ("error out"=w288:errorcluster)  [unwired: 12 in, 1 out]
        n106 = call-dynamic "destroy.vi"("abstract_vector_base in"=w284, "error in (no error)"=w288) -> ("error out"=w287:errorcluster)  [unwired: 12 in, 1 out]
        n107 = call-dynamic "destroy.vi"("error in (no error)"=w287, "abstract_llm_base in"=w283) -> ("error out"=w286:errorcluster)  [unwired: 8 in, 1 out]
        n108 = call-dynamic "destroy.vi"("error in (no error)"=w286, "abstract_llm_base in"=w282) -> ("error out"=w285:errorcluster)  [unwired: 8 in, 1 out]
        n109 = call <vilib>:"Add State(s) to Queue__jki_lib_state_machine.vi"("State(s) in (\"\")"=w293) -> ("States Out"=w292:string)  [unwired: 14 in]
      }
      frame "Agent: Ask" {
        n110 = Unbundle By Name(w299) -> ("Agent.last_message"=w296:refnum<class "message_text.lvclass">, "Agent.Agent_QA"=w302:refnum<class "agent_simple_qa.lvclass">)
        n111 = call-poly "ask_poly.vi"("error in (no error)"=w301, "message_text"=w296, "agent_simple_qa in"=w302) -> ("error out"=w300:errorcluster, "message_text_response"=w295:refnum<class "message_text.lvclass">, "agent_simple_qa out"=w298:refnum<class "agent_simple_qa.lvclass">)  [unwired: 6 in]
        n112 = Bundle By Name(cluster=w299, "Agent.last_message"=w295, "Agent.Agent_QA"=w298) -> (w297:T3)
        n113 = call <vilib>:"Add State(s) to Queue__jki_lib_state_machine.vi"("State(s) in Front (\"\")"="UI: UpdateChatMessage" ("State(s) in Front (\"\")"), "State(s) in (\"\")"=w304) -> ("States Out"=w303:string)  [unwired: 13 in]
      }
    }
  }
